vi "set_channel_params.vi"(8 "error in (no error)":errorcluster, 10 "motech_set_value":T1={"voltage"=0.0, "current"=0.01, "channel"=enum."1"}, 11 "Motech-pps-1200 in":refnum<class "Motech-pps-1200.lvclass">) -> (0 "error out":errorcluster, 3 "Motech-pps-1200 out":refnum<class "Motech-pps-1200.lvclass">)   [LabVIEW 2017, in "Motech-pps-1200.lvclass"]
uses:
  Motech-pps-1200.lvclass
  subVI/motech_power_supply/types/motech_set_value_cluster.ctl
  subVI/motech_power_supply/types/channels_enum.ctl
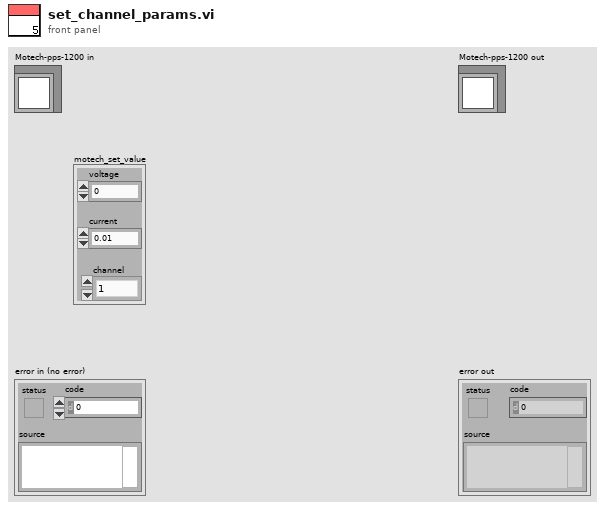
[diagram p1: front panel]
types:
  T1 = typedef "motech_set_value_cluster.ctl" = cluster{"voltage":dbl, "current":dbl, "channel":T2}
  T2 = typedef "channels_enum.ctl" = enum16{"0", "1", "2"}
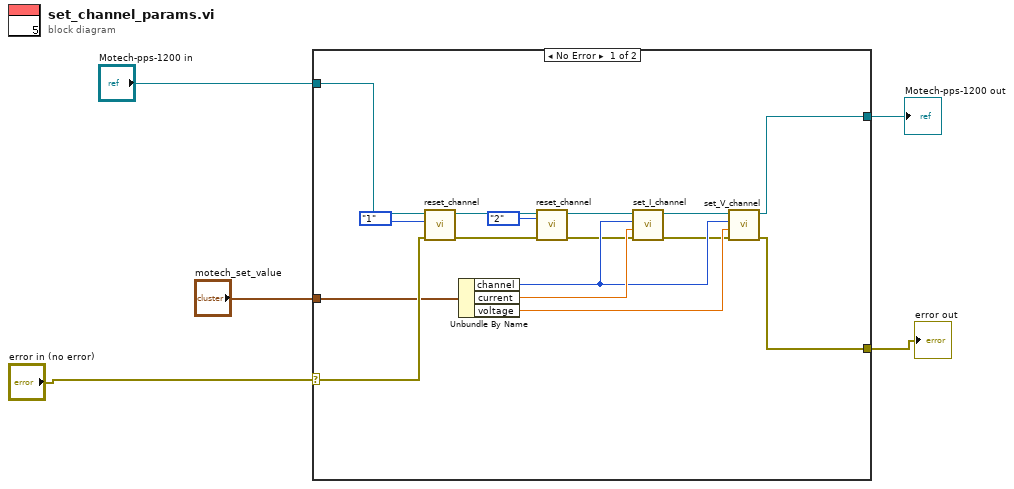
[diagram p0: block diagram]
diagram:
  n1 = case shown="No Error" "error in (no error)" {
    selector: "error in (no error)" -> [w17 w22]
    tunnel: "Motech-pps-1200 in" -> [w21 w23]
    tunnel: [w10 w23] -> w3
    tunnel: [w9 w22] -> w2
    tunnel: "motech_set_value" -> [w14 _]
    frame No Error {
      n2 = call "reset_channel.vi"("error in (no error)"=w17, "channel"=channels_enum."1", "Motech-pps-1200 in"=w21) -> ("error out"=w16:errorcluster, "Motech-pps-1200 out"=w20:refnum<class "Motech-pps-1200.lvclass">)  [unwired: 7 in]
      n3 = Unbundle By Name(w14) -> ("channel"=w11:T2, "current"=w13:dbl, "voltage"=w8:dbl)
      n4 = call "reset_channel.vi"("error in (no error)"=w16, "channel"=channels_enum."2", "Motech-pps-1200 in"=w20) -> ("error out"=w7:errorcluster, "Motech-pps-1200 out"=w15:refnum<class "Motech-pps-1200.lvclass">)  [unwired: 7 in]
      n5 = call-dynamic "set_I_channel.vi"("error in (no error)"=w7, "current"=w13, "channel"=w11, "Motech-pps-1200 in"=w15) -> ("error out"=w6:errorcluster, "Motech-pps-1200 out"=w12:refnum<class "Motech-pps-1200.lvclass">)  [unwired: 6 in]
      n6 = call-dynamic "set_V_channel.vi"("error in (no error)"=w6, "voltage"=w8, "channel"=w11, "Motech-pps-1200 in"=w12) -> ("error out"=w9:errorcluster, "Motech-pps-1200 out"=w10:refnum<class "Motech-pps-1200.lvclass">)  [unwired: 6 in]
    }
    frame Error {
    }
  }
  "error out" <- w2
  "Motech-pps-1200 out" <- w3
